vi "Untitled 1.vi"   [LabVIEW 2019]
uses:
  AD2_SDK_class/AD2_SDK.lvclass
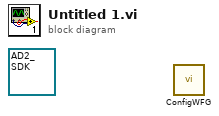
[diagram p0: block diagram]
diagram:
  (unwired) refnum<class "AD2_SDK.lvclass"> refnum ("AD2_SDK")
  n1 = call-dynamic "ConfigWFG.vi"() -> ()  [unwired: 18 in, 2 out]
